vi "count_up.vi"() -> ()   [LabVIEW 2020]
panel:
  out "num_iterations":i32
  in  "stop_button":bool
  out "is_running":bool
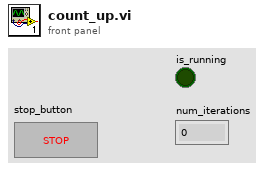
[diagram p1: front panel]
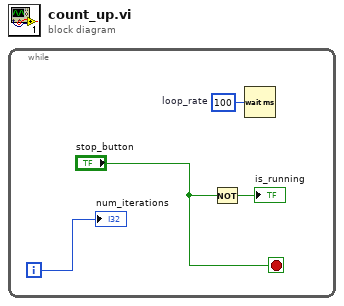
[diagram p0: block diagram]
diagram:
  n1 = while {
    i -> [w1]
    stop <- "stop_button" stop-if-true
    w3 = u32 100  # loop_rate
    n2 = Not(x="stop_button") -> (.not. x?=→"is_running":bool)
    n3 = Wait (ms)(milliseconds to wait=w3) -> ()  [unwired: 1 out]
    "num_iterations" <- w1
  }
